vi "Measurement Pass or Fail Decision.vi"(0 "Spec Values":T1(array[cluster]), 9 "Result data in":T2={"Measurement Names Array"=[], "Pass-Fail Array"=[], "Measurement Values Array "=[], "Roi for overlay (Arrows) Array"=[], "Algo Type Array"=[], "Image Array"=[], "Clamp operations"=enum."Average Clamp", "  Search Direction "=[], "Images_Array_in"=[], "ResultPF"=FALSE, "Total Cluster Values"={"Total Fail"=0, "Total Pass"=0, "Total Count"=0}, "Reel Counter Cluster"={"Reel Fail"=0, "Reel Pass"=0, "Reel Count"=0}, "Tolerance  Array"=[], "Array of Cam Spec Control Bool"=[], "Control Pass Fail Array"=[], "Specification Pass Fail Array"=[], "Overlay Arrow Lines"=[], "Camera ID"=[], "Trigger count"=0, "Specification fail?"=FALSE}, 11 "error in":errorcluster) -> (10 "Result data out":T2={"Measurement Names Array"=[], "Pass-Fail Array"=[], "Measurement Values Array "=[], "Roi for overlay (Arrows) Array"=[], "Algo Type Array"=[], "Image Array"=[], "Clamp operations"=enum."Average Clamp", "  Search Direction "=[], "Images_Array_in"=[], "ResultPF"=FALSE, "Total Cluster Values"={"Total Fail"=0, "Total Pass"=0, "Total Count"=0}, "Reel Counter Cluster"={"Reel Fail"=0, "Reel Pass"=0, "Reel Count"=0}, "Tolerance  Array"=[], "Array of Cam Spec Control Bool"=[], "Control Pass Fail Array"=[], "Specification Pass Fail Array"=[], "Overlay Arrow Lines"=[], "Camera ID"=[], "Trigger count"=0, "Specification fail?"=FALSE}, 15 "error Out":errorcluster)   [LabVIEW 2019, in "Algorithm.lvclass"]
uses:
  FrameworkOverrides/Algorithm.lvclass
  Controls/Result Cluster.ctl
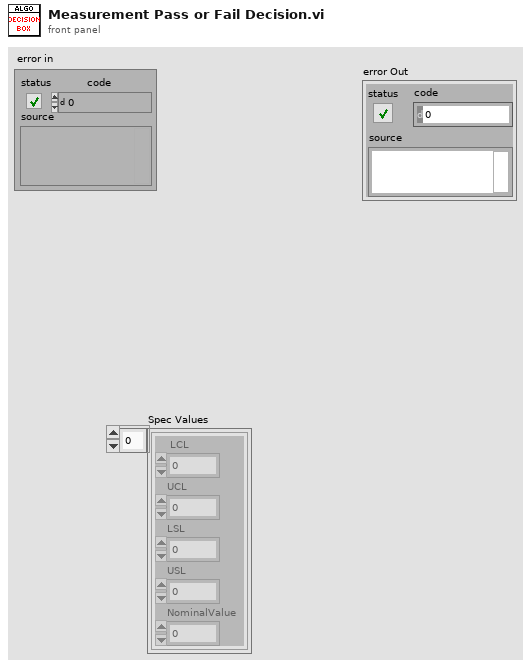
[diagram p1: front panel]
types:
  T1 = cluster{"LCL":dbl, "UCL":dbl, "LSL":dbl, "USL":dbl, "NominalValue":dbl}[]
  T2 = typedef "Algorithm.lvclass/Result Cluster.ctl" = cluster{"Measurement Names Array":string[], "Pass-Fail Array":bool[], "Measurement Values Array ":dbl[], "Roi for overlay (Arrows) Array":cluster{"Points for Arrow Overlay[0]":cluster{"x":dbl, "y":dbl}, "Points for Arrow Overlay[1]":cluster{"x":dbl, "y":dbl}, "Points for Arrow Overlay[2]":cluster{"x":dbl, "y":dbl}, "Points for Arrow Overlay[3]":cluster{"x":dbl, "y":dbl}}[], "Algo Type Array":string[], "Image Array":string[], "Clamp operations":enum16{"Min Clamp", "Max Clamp", "Average Clamp"}, "  Search Direction ":enum16{"Left to Right", "Right to Left", "Top to Bottom", "Bottom to Top"}[], "Images_Array_in":T3[], "ResultPF":bool, "Total Cluster Values":cluster{"Total Fail":u64, "Total Pass":u64, "Total Count":u64}, "Reel Counter Cluster":cluster{"Reel Fail":u64, "Reel Pass":u64, "Reel Count":u64}, "Tolerance  Array":string[], "Array of Cam Spec Control Bool":cluster{"Specification Boolean":bool, "Control Boolean":bool, "Camera ID":i8}[], "Control Pass Fail Array":bool[], "Specification Pass Fail Array":bool[], "Overlay Arrow Lines":cluster{"First Overlay Line ":cluster{"Start Point":cluster{"X":sgl, "Y":sgl}, "Start Point":cluster{"X":sgl, "Y":sgl}}, "Second Overlay Line ":cluster{"Start Point":cluster{"X":sgl, "Y":sgl}, "Start Point":cluster{"X":sgl, "Y":sgl}}}[], "Camera ID":i8[], "Trigger count":i32, "Specification fail?":bool}
  T3 = typedef "IMAQ Image.ctl" = refnum<image>
  T4 = cluster{"Specification Boolean":bool, "Control Boolean":bool, "Camera ID":i32}
  T5 = cluster{"LCL":string, "UCL":string, "LSL":string, "USL":string, "NominalValue":string}
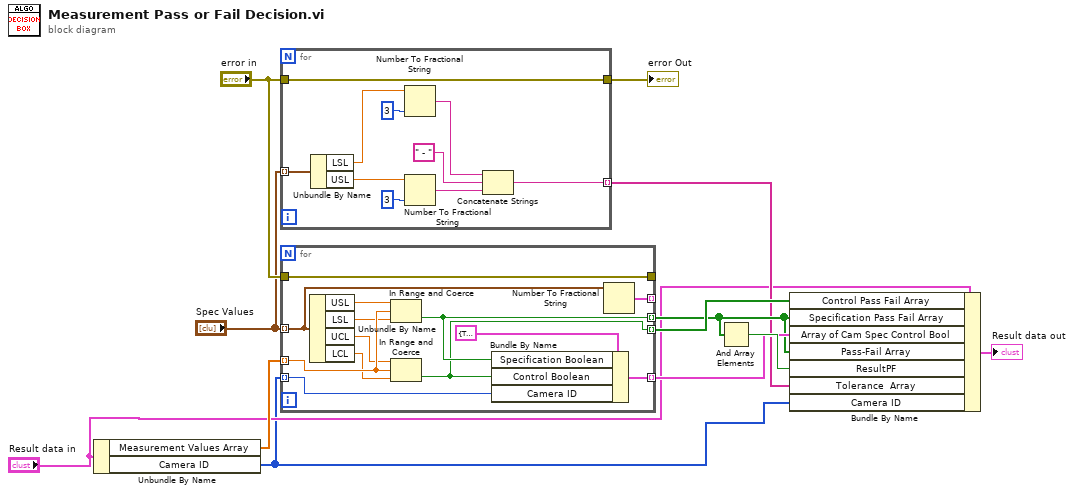
[diagram p0: block diagram]
diagram:
  n1 = Unbundle By Name("Result data in") -> ("Measurement Values Array"=w11:dbl[], "Camera ID"=w2:i8[])
  n2 = for {
    tunnel: "Spec Values" -> [w21] mode=indexing
    tunnel: [w14] -> w5 mode=indexing
    tunnel: "error in" -> [w13]
    tunnel: [w13] -> w1
    n3 = Unbundle By Name(w21) -> ("LSL"=w20:dbl, "USL"=w18:dbl)
    n4 = Number To Fractional String(number=w20, precision (6)=i16 3) -> (F-format string=w17:string)  [unwired: 2 in]
    n5 = Number To Fractional String(number=w18, precision (6)=i16 3) -> (F-format string=w15:string)  [unwired: 2 in]
    n6 = Concatenate Strings(w17, " - " ("string"), w15) -> (w14:string)
  }
  "error Out" <- w1
  n7 = for {
    tunnel: [w28] -> w7 mode=indexing
    tunnel: "error in" -> [w35]
    tunnel: [w27] -> w8 mode=indexing
    tunnel: [w35] -> _
    tunnel: w11 -> [w34] mode=indexing
    tunnel: "Spec Values" -> [w24] mode=indexing
    tunnel: w2 -> [w26] mode=indexing
    tunnel: [w25] -> w9 mode=indexing
    tunnel: [w23] -> _ mode=indexing
    n8 = Unbundle By Name(w24) -> ("USL"=w33:dbl, "LSL"=w32:dbl, "UCL"=w31:dbl, "LCL"=w30:dbl)
    n9 = In Range and Coerce(upper limit=w33, x=w34, lower limit=w32) -> (In Range?=w28:bool)  [unwired: 1 out]
    n10 = In Range and Coerce(upper limit=w31, x=w34, lower limit=w30) -> (In Range?=w27:bool)  [unwired: 1 out]
    n11 = Bundle By Name(cluster=T4 {"Specification Boolean"=TRUE, "Control Boolean"=TRUE, "Camera ID"=0}, "Specification Boolean"=w28, "Control Boolean"=w27, "Camera ID"=w26) -> (w25:T4)
    n12 = Number To Fractional String(number=w24) -> (F-format string=w23:T5)  [unwired: 3 in]
  }
  n13 = And Array Elements(Boolean array=w7) -> (logical AND=w10:bool)
  n14 = Bundle By Name(cluster="Result data in", "Control Pass Fail Array"=w8, "Specification Pass Fail Array"=w7, "Array of Cam Spec Control Bool"=w9, "Pass-Fail Array"=w7, "ResultPF"=w10, "Tolerance  Array"=w5, "Camera ID"=w2) -> (→"Result data out":T2)
